vi "Run3.vi"() -> ()   [LabVIEW 2015]
uses:
  <vilib>/NXT/LegoClasses/BrickReference/BrickReference.lvclass
  <vilib>/NXT/Subs/LVHSConnector.ctl
panel:
  in  "NXT/EV3":T1
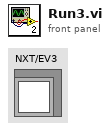
[diagram p1: front panel]
types:
  T1 = typedef "LVHSConnector.ctl" = refnum<class "BrickReference.lvclass">
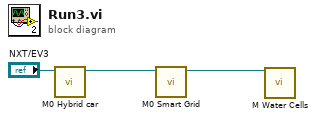
[diagram p0: block diagram]
diagram:
  n1 = call "M0 Hybrid car.vi"("NXT/EV3"="NXT/EV3") -> ("EV3 out"=w3:T1)  [unwired: 10 in]
  n2 = call "M0 Smart Grid.vi"("EV3 in"=w3) -> ("EV3 out"=w1:T1)  [unwired: 10 in]
  n3 = call "M Water Cells.vi"("EV3 in"=w1) -> ()  [unwired: 11 in]
